vi "PDC_DetectDevice.vi"(0 "InterfaceCode":u32, 5 "DetectNum":u32, 7 "DetectParam":u32, 11 "error in (no error)":errorcluster, 12 "DetectNo":u32[](array[numeric])) -> (3 "DeviceNum":u32, 4 "ReturnValue":u32, 6 "DeviceCode":u32[](array[numeric]), 8 "TmpDeviceNo":u32[](array[numeric]), 10 "InterfaceCode(out)":u32[](array[numeric]), 14 "ErrorCode":u32, 15 "error out":errorcluster)   [LabVIEW 2015]
doc: "This VI searches for devices that can be opened and retrieves the number of those devices."
uses:
  PDCLIB.dll
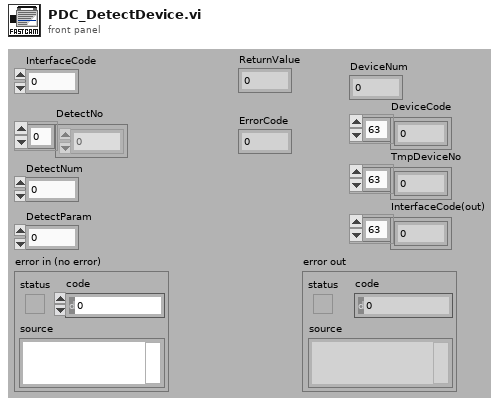
[diagram p1: front panel]
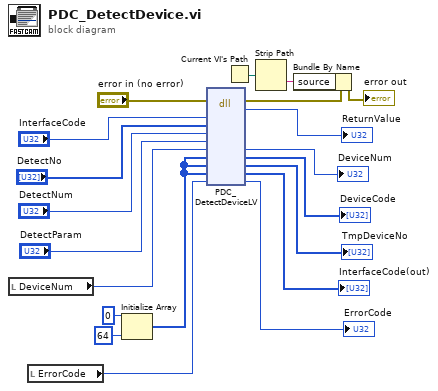
[diagram p0: block diagram]
diagram:
  n1 = local read "DeviceNum"() -> (w6:u32)
  n2 = local read "ErrorCode"() -> (w18:u32)
  n3 = Initialize Array(u32 0 ("—v‘f"), 64 ("dimension size")) -> (w7:u32[])
  n4 = dll-call lib="PDCLIB.dll" fn="PDC_DetectDeviceLV"(error in="error in (no error)", "nInterfaceCode"="InterfaceCode", "pDetectNo"="DetectNo", "nDetectNum"="DetectNum", "nDetectParam"="DetectParam", "m_nDeviceNum"=w6, "m_nDeviceCode"=w7, "m_nTmpDeviceNo"=w7, "m_nInterfaceCode"=w7, "pErrorCode"=w18) -> (error out=w10:errorcluster, "return type"=→"ReturnValue":u32, "m_nDeviceNum"=→"DeviceNum":u32, "m_nDeviceCode"=→"DeviceCode":u32[], "m_nTmpDeviceNo"=→"TmpDeviceNo":u32[], "m_nInterfaceCode"=→"InterfaceCode(out)":u32[], "pErrorCode"=→"ErrorCode":u32)  [unwired: 6 in, 1 out]
  n5 = Current VI's Path() -> (path=w11:path)
  n6 = Strip Path(path=w11) -> (name=w12:string)  [unwired: 1 out]
  n7 = Bundle By Name(cluster=w10, "source"=w12) -> (→"error out":errorcluster)
